vi "InitDataComms.vi"(8 "error in (no error)":errorcluster, 11 "C37.118 PMU in":refnum<class "C37.118 PMU.lvclass">) -> (0 "error out":errorcluster, 3 "C37.118 PMU out":refnum<class "C37.118 PMU.lvclass">)   [LabVIEW 2018, in "SensorPlugins.lvlib" / "C37.118 PMU.lvclass"]
uses:
  C37.118 PMU.lvclass
  C37.118 PMU.lvclass/C37.118 PMU.ctl
  <userlib>/NIST/Socket Class/Classes/Socket.Base/Socket.Base.lvclass/Socket.Base.ctl
  <userlib>/NIST/Socket Class/Classes/Socket.Base/Socket.Base.lvclass
  <userlib>/NIST/Socket Class/Classes/Socket.TCP/Socket.TCP.lvclass
  C:/Program Files/National Instruments/LabVIEW 2018/user.lib/NIST/Socket Class/Classes/Socket.Base/Socket.Base.lvclass
  <userlib>/NIST/Socket Class/Classes/Socket.UDP/Socket.UDP.lvclass
  Accessors/Write DataSocket.vi
  Accessors/Read DataSocket.vi
  Accessors/Read PMUComms.vi
  <userlib>/NIST/Socket Class/Classes/Socket.Base/Accessors/Read initialized.vi
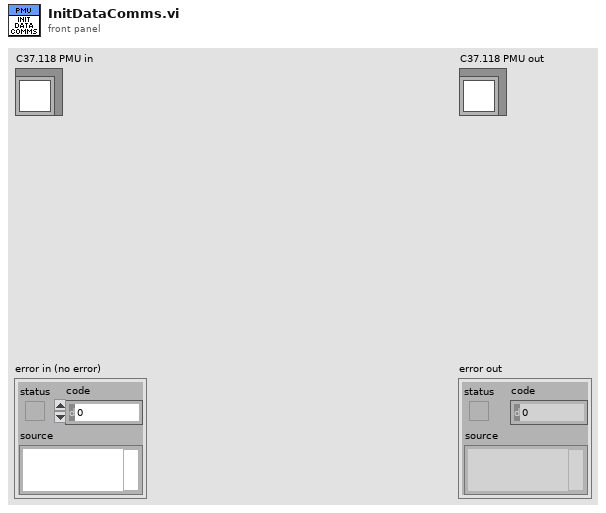
[diagram p1: front panel]
types:
  T1 = typedef "SensorPlugins.lvlib/C37.118 PMU.lvclass/PMUComms.ctl" = cluster{"PMU IP Address":string, "CMD Comms Type":T2, "Data Comms Type":T2, "CMD Port":u16, "Data Port":u16, "PMU ID":u16}
  T2 = typedef "SensorPlugins.lvlib/C37.118 PMU.lvclass/eCommsType.ctl" = enum16{"TCP", "UDP", "USB", "GPIB"}
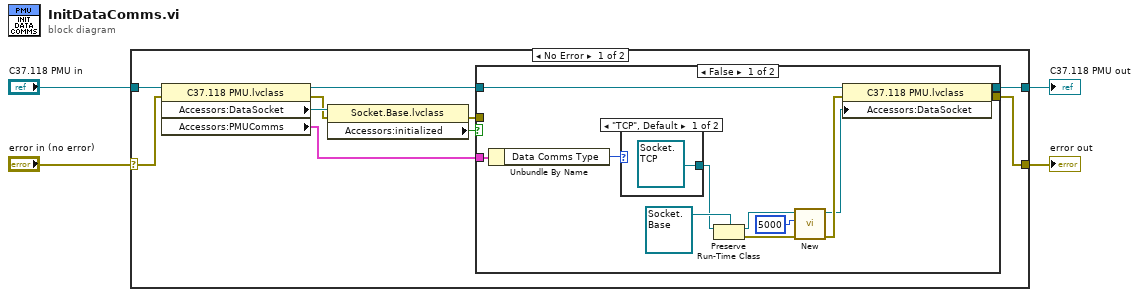
[diagram p0: block diagram]
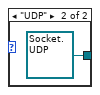
[diagram p2: hidden frame]
diagram:
  n1 = case shown="No Error" "error in (no error)" {
    selector: "error in (no error)" -> [w13 w32]
    tunnel: [w11 w32] -> w3
    tunnel: [w10 w31] -> w1
    tunnel: "C37.118 PMU in" -> [w14 w31]
    frame No Error {
      n2 = property class="C37.118 PMU.lvclass"(reference=w14, error in=w13) -> (reference out=w12:refnum<class "C37.118 PMU.lvclass">, error out=w8:errorcluster, "Accessors:DataSocket"=w9:refnum<class "Socket.Base.lvclass">, "Accessors:PMUComms"=w7:T1)
      n3 = property class="Socket.Base.lvclass"(reference=w9, error in=w8) -> (error out=w6:errorcluster, "Accessors:initialized"=w5:bool)  [unwired: 1 out]
      n4 = case shown="False" w5 {
        tunnel: w12 -> [w25 w30]
        tunnel: [w24 w29] -> w11
        tunnel: [w23 w30] -> w10
        tunnel: w7 -> [w15 _]
        tunnel: w6 -> [_ w29]
        frame False {
          n5 = Unbundle By Name(w15) -> ("Data Comms Type"=w26:T2)
          n6 = case shown="\"TCP\", Default" w26 {
            tunnel: [refnum<class "Socket.TCP.lvclass"> refnum ("Socket.TCP in") refnum<class "Socket.UDP.lvclass"> refnum ("Socket.UDP in")] -> w16
            frame "TCP", Default {
            }
            frame "UDP" {
            }
          }
          n7 = Preserve Run-Time Class(object in=w16, 2:refnum<class "Socket.Base.lvclass"> refnum ("Socket.Base in")) -> (object out=w22:refnum<class "Socket.Base.lvclass">, error out=w21:errorcluster)  [unwired: 1 in]
          n8 = call-dynamic "New.vi"("error in (no error)"=w21, "timeout"=5000, "Socket.Base in"=w22) -> ("error out"=w20:errorcluster, "Socket.Base out"=w19:refnum<class "Socket.Base.lvclass">)  [unwired: 7 in]
          n9 = property class="C37.118 PMU.lvclass"(reference=w25, error in=w20, "Accessors:DataSocket"=w19) -> (reference out=w23:refnum<class "C37.118 PMU.lvclass">, error out=w24:errorcluster)
        }
        frame True {
        }
      }
    }
    frame Error {
    }
  }
  "error out" <- w3
  "C37.118 PMU out" <- w1
